vi "maxabs_scales.vi"(8 "error in":errorcluster caption="entrée d'erreur", 10 "X":string[][](array[string]), 11 "maxabs_scale":cluster{"axis":i32, "copy":bool}={"axis"=0, "copy"=TRUE}) -> (0 "error out":errorcluster caption="sortie d'erreur", 3 "Data":T1)   [LabVIEW 2020]
doc: "Scale each feature to the [-1, 1] range without breaking the sparsity.\n\nThis estimator scales each feature individually such that the maximal absolute value of each feature in the training set will be 1.0.\n\nThis scaler can also be applied to sparse CSR or CSC matrices.\n\nParameters :\n\n- X : array-like, shape (n_samples, n_features)\nThe data.\n\n- axis : int (0 by default)\naxis used to scale along. If 0, independently scale each feature, otherwise (if 1) scale each sample.\n\n- copy : boolean, optional, default is True\nSet to False to perform inplace scaling and avoid a copy (if the input is already a numpy array)."
uses:
  maxabs_scale.lvclass
panel:
  out "maxabs_scale.lvclass":refnum<class "maxabs_scale.lvclass">
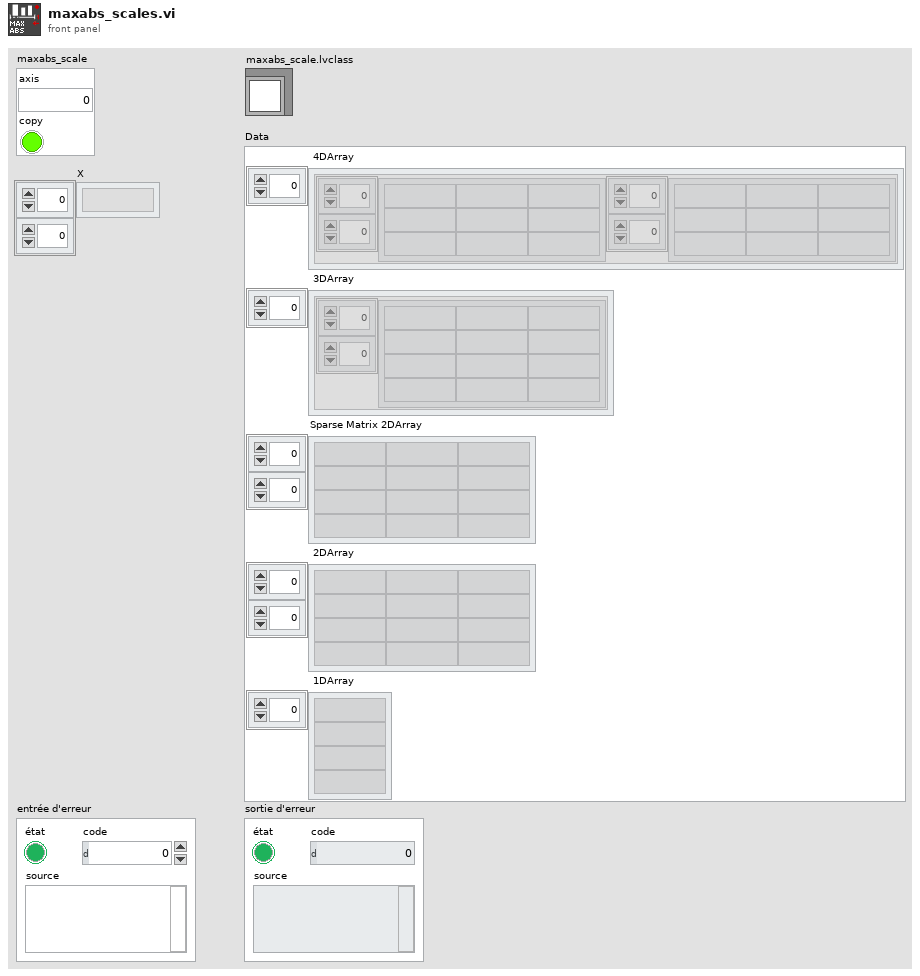
[diagram p1: front panel]
types:
  T1 = cluster{" 4DArray":cluster{"1":string[][], "2":string[][]}[], " 3DArray":cluster{"Tableau":string[][]}[], "Sparse Matrix 2DArray":string[][], " 2DArray":string[][], " 1DArray":string[]}
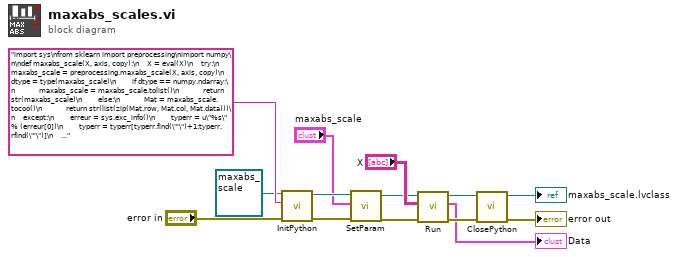
[diagram p0: block diagram]
diagram:
  n1 = call-dynamic "InitPython.vi"("error in (no error)"="error in", "Python Instruction"="import sys\nfrom sklearn import preprocessing\nimport numpy\n\ndef maxabs_scale(X, axis, copy):\n    X = eval(X)\n    try:\n        maxabs_scale = preprocessing.maxabs_scale(X, axis, copy)\n        dtype = type(maxabs_scale)\n        if dtype == numpy.ndarray:\n            maxabs_scale = maxabs_scale.tolist()\n            return str(maxabs_scale)\n        else:\n            Mat = maxabs_scale.tocoo()\n            return str(list(zip(Mat.row, Mat.col, Mat.data)))\n    except:\n        erreur = sys.exc_info()\n        typerr = u\"%s\" % (erreur[0])\n        typerr = typerr[typerr.find(\"'\")+1:typerr.rfind(\"'\")]\n        msgerr = u\"%s\" % (erreur[1])\n        message = str('/!\\\\ {0} : {1}'. format(typerr,msgerr))\n        return message", "Scikit-learn en entrée"=refnum<class "maxabs_scale.lvclass"> refnum ("maxabs_scale.lvclass")) -> ("error out"=w8:errorcluster, "Scikit-learn en sortie"=w10:refnum<class "maxabs_scale.lvclass">)  [unwired: 7 in]
  n2 = call-dynamic "SetParam.vi"("error in (no error)"=w8, "maxabs_scale"="maxabs_scale", "maxabs_scale.lvclass"=w10) -> ("error out"=w5:errorcluster, "maxabs_scale.lvclass"=w6:refnum<class "maxabs_scale.lvclass">)  [unwired: 7 in]
  n3 = call-dynamic "Run.vi"("error in (no error)"=w5, "X"="X", "maxabs_scale.lvclass"=w6) -> ("error out"=w3:errorcluster, "Data"=→"Data":T1, "maxabs_scale.lvclass"=w4:refnum<class "maxabs_scale.lvclass">)  [unwired: 6 in]
  n4 = call-dynamic "ClosePython.vi"("error in (no error)"=w3, "Scikit-learn en entrée"=w4) -> ("error out"=→"error out":errorcluster, "Scikit-learn en sortie"=→"maxabs_scale.lvclass":refnum<class "maxabs_scale.lvclass">)  [unwired: 8 in]
